vi "Calc K Error.vi"(7 "Reobserved Array":bool[](array[boolean]), 8 "Error In":errorcluster, 10 "SLAM In":T1) -> (0 "error out":errorcluster, 2 "SLAM Out":T1, 5 "Reobserved Array Out":bool[](array[boolean]))   [LabVIEW 2009]
uses:
  Controls/SLAM.ctl
  <vilib>/Analysis/Matrix/Datatypes/RealMatrix.ctl
  <vilib>/Analysis/Matrix/NI_Matrix.lvlib
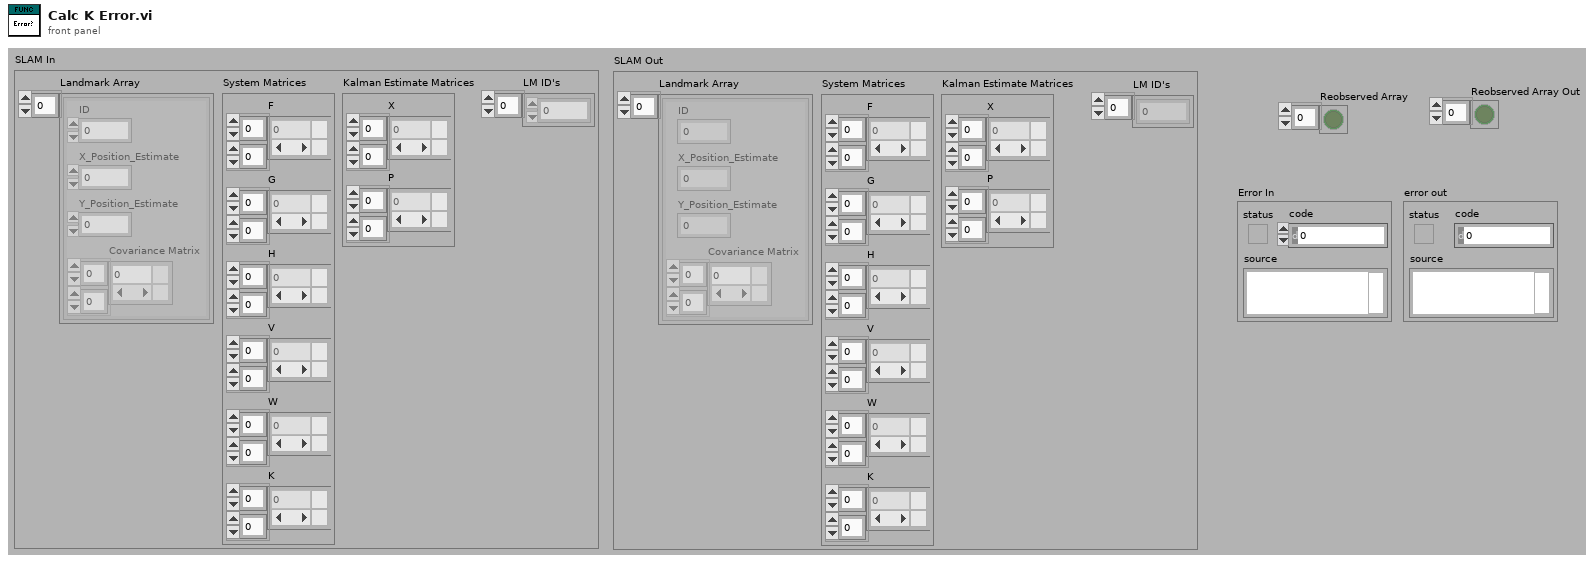
[diagram p1: front panel]
types:
  T1 = typedef "SLAM.ctl" = cluster{"Landmark Array":cluster{"ID":dbl, "X_Position_Estimate":dbl, "Y_Position_Estimate":dbl, "Covariance Matrix":T2}[], "System Matrices":cluster{"F":T2, "G":T2, "H":T2, "V":T2, "W":T2, "K":T2}, "Kalman Estimate Matrices":cluster{"X":T2, "P":T2}, "LM ID's":dbl[]}
  T2 = typedef "NI_Matrix.lvlib/RealMatrix.ctl" = dbl[][]
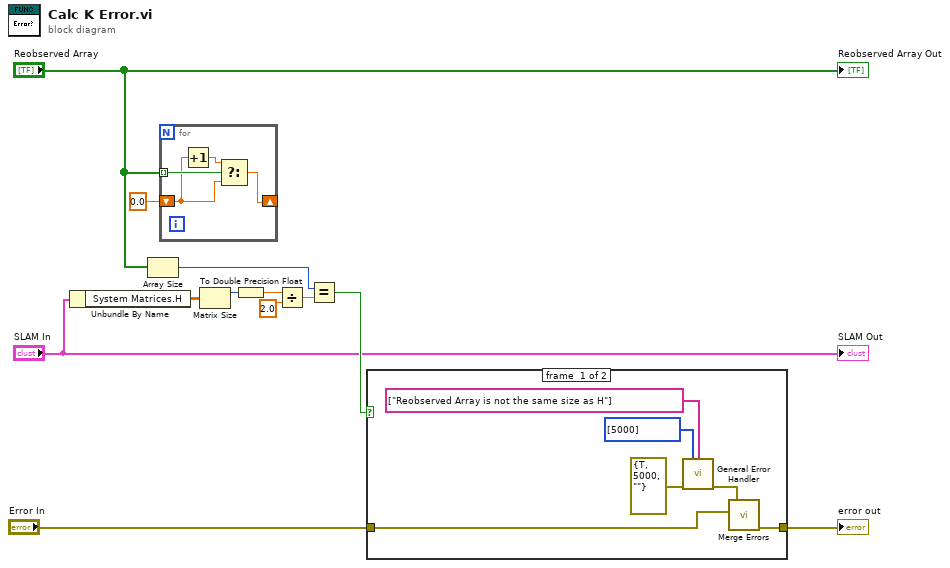
[diagram p0: block diagram]
diagram:
  n1 = Unbundle By Name("SLAM In") -> ("System Matrices.H"=w7:T2)
  n2 = Array Size(array="Reobserved Array") -> (size(s)=w1:i32)
  n3 = for {
    tunnel: "Reobserved Array" -> [w16] mode=indexing
    shift-right: [w15] -> _
    shift-left: 0.0 ("y") -> [w13]
    n4 = Increment(x=w13) -> (x+1=w14:dbl)
    n5 = Select(t=w14, s=w16, f=w13) -> (s? t:f=w15:dbl)
  }
  n6 = Matrix Size(0:w7) -> (1:w9:i32)  [unwired: 1 out]
  n7 = To Double Precision Float(number=w9) -> (double precision float=w11:dbl)
  n8 = Divide(x=w11, y=2.0) -> (x/y=w8:dbl)
  n9 = Equal?(x=w1, y=w8) -> (x = y?=w12:bool)
  n10 = case shown="False" w12 {
    tunnel: [w18 w23] -> w5
    tunnel: "Error In" -> [w17 w23]
    frame #0 {
      n11 = call <vilib>:"General Error Handler.vi"("[user-defined codes]"=i32[] [5000], "[user-defined descriptions]"=string[] ["Reobserved Array is not the same size as H"], "error in (no error)"=errorcluster {"status"=TRUE, "code"=5000, "source"=""}) -> ("error out"=w19:errorcluster)  [unwired: 8 in, 4 out]
      n12 = call <vilib>:"Merge Errors.vi"("error in 2 (no error)"=w17, "error in 1 (no error)"=w19) -> ("error out"=w18:errorcluster)  [unwired: 5 in]
    }
    frame #1 {
    }
  }
  "error out" <- w5
  "Reobserved Array Out" <- "Reobserved Array"
  "SLAM Out" <- "SLAM In"
